vi "Day01-2.vi"() -> ()   [LabVIEW 2021]
panel:
  out "sum":i16
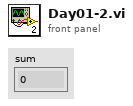
[diagram p1: front panel]
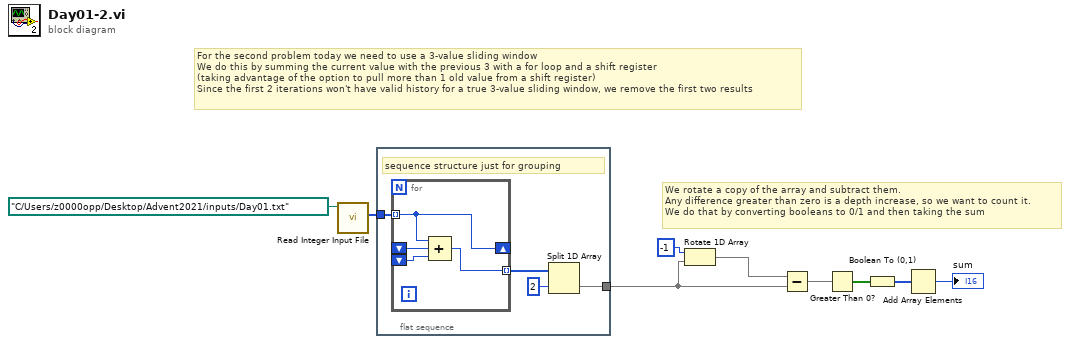
[diagram p0: block diagram]
diagram:
  # "For the second problem today we need to use a 3-value sliding window\nWe do this by summing the current value with the previous 3 with a for loop and a shift register\n(taking advantage of the option to pull more than 1 old value from a shift register)\nSince the first 2 iterations won't have valid history for a true 3-value sliding window, we remove the first two results"
  # "We rotate a copy of the array and subtract them.\nAny difference greater than zero is a depth increase, so we want to count it.\nWe do that by converting booleans to 0/1 and then taking the sum"
  n1 = call "Read Integer Input File.vi"("file path (dialog if empty)"=path "C:/Users/z0000opp/Desktop/Advent2021/inputs/Day01.txt") -> ("input values"=w2:i64[])  [unwired: 10 in]
  n2 = flat-sequence {
    tunnel: w2 -> [w11]
    tunnel: [w10] -> w1
    frame #0 {
      # "sequence structure just for grouping"
      n3 = for {
        tunnel: w11 -> [w15] mode=indexing
        shift-right: [w15] -> _
        shift-left: _ -> [w17]
        shift-left: _ -> [w16]
        tunnel: [w14] -> w13 mode=indexing
        n4 = Compound Arithmetic op=ADD(w15, w17, w16) -> (w14:i64)
      }
      n5 = Split 1D Array(array=w13, index=2) -> (second subarray=w10:i64[])  [unwired: 1 out]
    }
  }
  n6 = Rotate 1D Array(1:w1, 2:-1 ("n")) -> (0:w8:i64[])
  n7 = Subtract(x=w8, y=w1) -> (x-y=w6:i64[])
  n8 = Greater Than 0?(x=w6) -> (x > 0?=w5:bool[])
  n9 = Boolean To (0,1)(Boolean=w5) -> (0, 1=w4:i16[])
  n10 = Add Array Elements(numeric array=w4) -> (sum=→"sum":i16)
